vi "MessagerAccepted.vi"(10 "id":string) -> ()   [LabVIEW 2018]
panel:
  out "String":string
  # "EN UN MOMENTO UN EMPLEADO DE BBVA SE\nPONDRA EN CONTACTO CONTIGO."
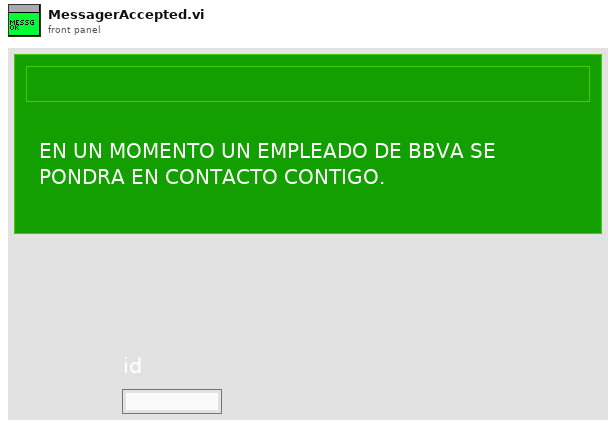
[diagram p1: front panel]
types:
  T1 = enum32{"Invalid", "Standard", "Closed", "Hidden", "Minimized", "Maximized"}
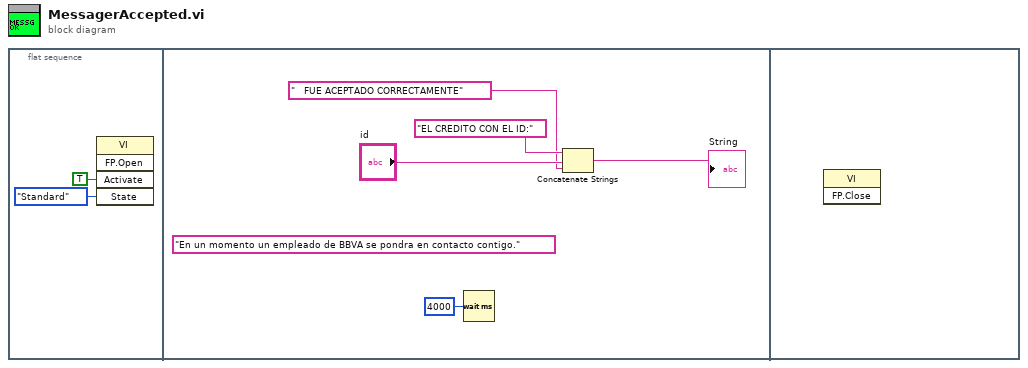
[diagram p0: block diagram]
diagram:
  n1 = flat-sequence {
    frame #0 {
      n2 = invoke class="VI" method="FP.Open"("Activate"=TRUE ("Activate?"), "State"=T1."Standard") -> ()  [unwired: 3 in, 5 out]
    }
    frame #1 {
      (unwired) "En un momento un empleado de BBVA se pondra en contacto contigo." ("string")
      n3 = Wait (ms)(milliseconds to wait=u32 4000) -> ()  [unwired: 1 out]
      n4 = Concatenate Strings("EL CREDITO CON EL ID:" ("string"), "id", "   FUE ACEPTADO CORRECTAMENTE" ("string")) -> (→"String":string)
    }
    frame #2 {
      n5 = invoke class="VI" method="FP.Close"() -> ()  [unwired: 3 in, 3 out]
    }
  }
